vi "Write to Observer.vi"(8 "error in":errorcluster, 11 "tCRD in":refnum<class "Aircraft OPCCRD.lvclass">) -> (0 "error out":errorcluster, 3 "tCRD out":refnum<class "Aircraft OPCCRD.lvclass">)   [LabVIEW 2015, in "Aircraft OPCCRD.lvclass"]
uses:
  Aircraft OPCCRD.lvclass
  Aircraft OPCCRD.lvclass/Aircraft OPCCRD.ctl
  Reusable/File IO/Class/File Observer.lvclass
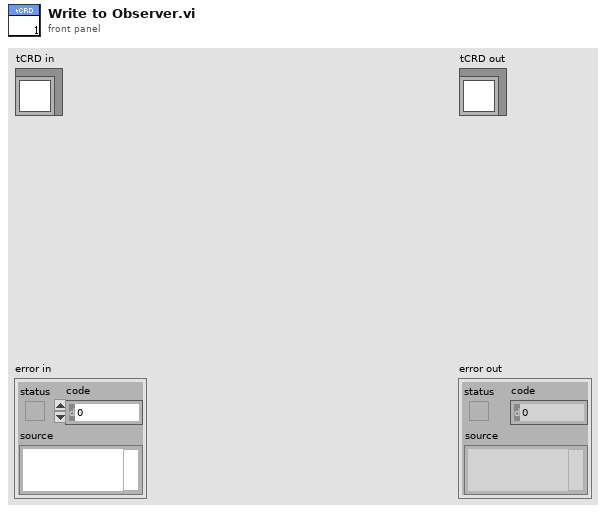
[diagram p1: front panel]
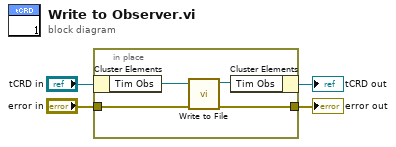
[diagram p0: block diagram]
diagram:
  n1 = in-place {
    in-place-border: "error in" -> [w6]
    in-place-border: [w5] -> w3
    n2 = in-place-cluster #1("tCRD in") -> ("Tim Obs"=w8:refnum<class "Tim File Observer.lvclass">)
    n3 = call "Write to File.vi"("error in"=w6, "File Obs in"=w8) -> ("error out"=w5:errorcluster, "File Obs out"=w7:refnum<class "Tim File Observer.lvclass">)  [unwired: 8 in]
    n4 = in-place-cluster #1("Tim Obs"=w7) -> (→"tCRD out":refnum<class "Aircraft OPCCRD.lvclass">)
  }
  "error out" <- w3
